vi "LIA_Host_FloatingPoint.vi"() -> ()   [LabVIEW 2012]
uses:
  <vilib>/userdefined/High Color/nirio_resource_hc.ctl
  <vilib>/LabVIEW Targets/FPGA/cRIO/shared/nicrio_ModuleControls/nicrio_cRIO-9233_DataRatesRing.ctl
  <vilib>/FPGAPlugInAG/PCI-7831R/niLvFpga_Open_PCI-7831R.vi
  <vilib>/FPGAPlugInAG/PCI-7831R/niLvFpga_Download_PCI-7831R.vi
  <vilib>/FPGAPlugInAG/PCI-7831R/niLvFpga_Reset_PCI-7831R.vi
  <vilib>/Utility/error.llb/Error Cluster From Error Code.vi
  <vilib>/FPGAPlugInAG/PCI-7831R/niLvFpga_Run_PCI-7831R.vi
  <vilib>/RVI Host/nirviSupport.llb/nirviErrorClusterFromErrorCode.vi
  <vilib>/rvi/errors/niLvFpgaAdjustHostInterfaceError.vi
  <vilib>/FPGAPlugInAG/PCI-7831R/niLvFpga_Close_PCI-7831R.vi
  <vilib>/rvi/interface/nirviOpenFPGA/nirviOpenFPGA.xnode
  FPGA Bitfiles/LIA_FPGATarget_LIAFPGA_UBXKlbf10UU.lvbitx
  LIA_FPGA.vi
  <vilib>/rvi/interface/nirviMethod/nirviMethod.xnode
  <vilib>/rvi/interface/nirviReadWriteControl/nirviReadWriteControl.xnode
  <vilib>/rvi/interface/nirviCloseFPGA/nirviCloseFPGA.xnode
  <vilib>/rvi/errors/niLvFpgaMergeErrorWithErrorCode.vi
  <vilib>/FPGAPlugInAG/PCI-7831R/niLvFpga_ConfigureFifo_PCI-7831R.vi
  <vilib>/rvi/interface/nirviMethod/StockFPGA_InlinedMethodWaitForSingleIRQ.vi
  <vilib>/FPGAPlugInAG/PCI-7831R/niLvFpga_WaitOnIrq_PCI-7831R.vi
  <vilib>/FPGAPlugInAG/PCI-7831R/niLvFpga_AcknowledgeIrq_PCI-7831R.vi
  <vilib>/FPGAPlugInAG/PCI-7831R/niLvFpga_ReadFifo_PCI-7831R.vi
  NiFpgaLv.dll
panel:
  in  "Elements Remaining":u32
  in  "Offset":sgl
  in  "LSB Weight":sgl
  out "Locked?":bool
  out "Locked Frequency [Hz]":dbl
  out "Phase [degree]":dbl
  out "Amplitude [V]":dbl
  in  "Data Rate":T1=2 items=["50.000 kS/s (NI 9233)"=2, "33.333 kS/s (NI 9233)"=3, "25.000 kS/s (NI 9233)"=34, "16.667 kS/s (NI 9233)"=35, "12.500 kS/s (NI 9233)"=36, "10.000 kS/s (NI 9233)"=37, "  8.333 kS/s (NI 9233)"=38, "  7.143 kS/s (NI 9233)"=39, "  6.250 kS/s (NI 9233)"=40, "  5.556 kS/s (NI 9233)"=41, "  5.000 kS/s (NI 9233)"=42, "  4.545 kS/s (NI 9233)"=43, "  4.167 kS/s (NI 9233)"=44, "  3.846 kS/s (NI 9233)"=45, "  3.571 kS/s (NI 9233)"=46, "  3.333 kS/s (NI 9233)"=47, "  3.125 kS/s (NI 9233)"=48, "  2.941 kS/s (NI 9233)"=49, "  2.778 kS/s (NI 9233)"=50, "  2.632 kS/s (NI 9233)"=51, "  2.500 kS/s (NI 9233)"=52, "  2.381 kS/s (NI 9233)"=53, "  2.273 kS/s (NI 9233)"=54, "  2.174 kS/s (NI 9233)"=55, "  2.083 kS/s (NI 9233)"=56, "  2.000 kS/s (NI 9233)"=57]
  out "Waveform Graph":sgl[][](graph)
  in  "stop":bool
  out "channel Q":dbl
  out "channel I":dbl
  in  "Filter Rolloff":enum16{"20 dB", "40 dB", "60 dB", "80 dB"}(ring)
  in  "Time Constant [s]":dbl=1.0 format="%.2f"
  in  "Resource Name":T2
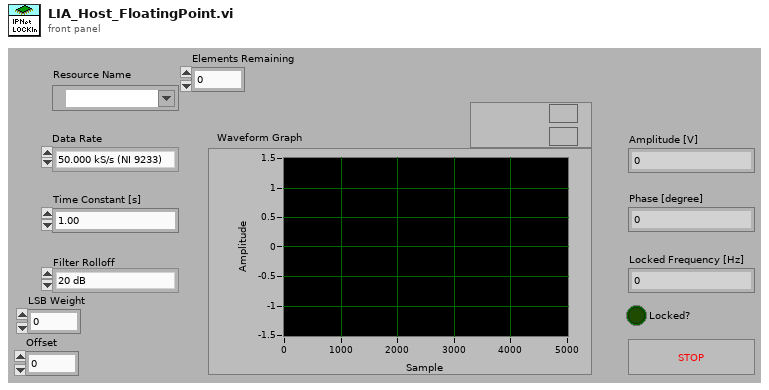
[diagram p1: front panel]
types:
  T1 = typedef "nicrio_cRIO-9233_DataRatesRing.ctl" = u8
  T2 = typedef "nirio_resource_hc.ctl" = tag
  T3 = enum16{"Reserved", "Sine", "Square", "Sine (sync)"}
  T4 = cluster{"fr":dbl, "Phase":dbl, "Order":u32, "Updated":bool, "Block Size":i32, "fs":dbl}
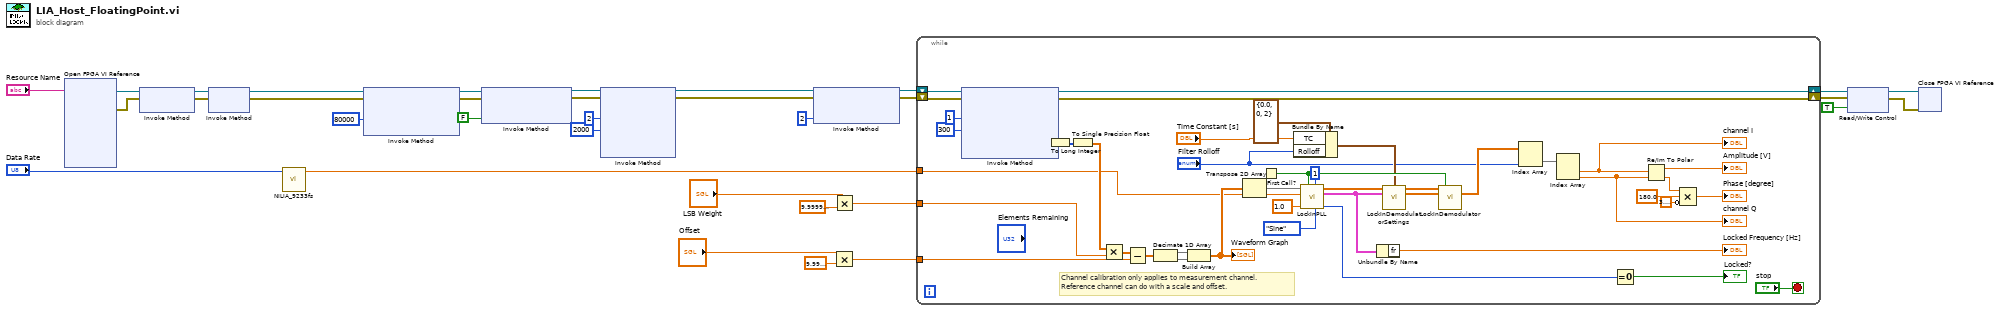
[diagram p0: block diagram]
diagram:
  n1 = xnode "Open FPGA VI Reference"("resource name"="Resource Name") -> ("FPGA VI Reference Out"=w33:refnum<k20>, "error out"=w32:errorcluster)  [unwired: 1 in]
  n2 = xnode "Invoke Method"("FPGA VI Reference In"=w33, "error in"=w32) -> ("FPGA VI Reference Out"=w31:refnum<k20>, "error out"=w30:errorcluster)
  n3 = xnode "Invoke Method"("FPGA VI Reference In"=w31, "error in"=w30) -> ("FPGA VI Reference Out"=w6:refnum<k20>, "error out"=w5:errorcluster)
  n4 = call "NILIA_9233fs.vi"("Data Rate"="Data Rate") -> ("fs"=w7:dbl)  [unwired: 10 in]
  n5 = xnode "Invoke Method"("FPGA VI Reference In"=w6, "error in"=w5, "Requested Depth"=u32 80000 ("Depth")) -> ("FPGA VI Reference Out"=w22:refnum<k20>, "error out"=w21:errorcluster)  [unwired: 1 out]
  n6 = xnode "Invoke Method"("FPGA VI Reference In"=w22, "error in"=w21, "Wait Until Done (F)"=FALSE) -> ("FPGA VI Reference Out"=w27:refnum<k20>, "error out"=w26:errorcluster)
  n7 = xnode "Invoke Method"("FPGA VI Reference In"=w27, "error in"=w26, "IRQ Number(s)"=2, "Timeout (ms)"=2000) -> ("FPGA VI Reference Out"=w2:refnum<k20>, "error out"=w1:errorcluster)  [unwired: 2 out]
  n8 = xnode "Invoke Method"("FPGA VI Reference In"=w2, "error in"=w1, "IRQ Number(s)"=2) -> ("FPGA VI Reference Out"=w20:refnum<k20>, "error out"=w19:errorcluster)
  n9 = Multiply(x="Offset", y=sgl 1e-09) -> (x*y=w9:sgl)
  n10 = Multiply(x="LSB Weight", y=sgl 1e-12) -> (x*y=w17:sgl)
  n11 = while {
    shift-right: [w62] -> w16
    shift-left: w20 -> [w70]
    shift-right: [w61] -> w15
    shift-left: w19 -> [w69]
    tunnel: w17 -> [w67]
    tunnel: w9 -> [w68]
    tunnel: w7 -> [w46]
    stop <- "stop" stop-if-true
    # "Channel calibration only applies to measurement channel.\nReference channel can do with a scale and offset."
    n12 = xnode "Invoke Method"("FPGA VI Reference In"=w70, "error in"=w69, "Number of Elements"=u32 1, "Timeout (ms)"=300) -> ("FPGA VI Reference Out"=w62:refnum<k20>, "error out"=w61:errorcluster, "Data"=w72:i32[])  [unwired: 1 out]
    n13 = To Long Integer(number=w72) -> (32bit integer=w71:i32[])
    n14 = To Single Precision Float(number=w71) -> (single precision float=w66:sgl[])
    n15 = Multiply(x=w66, y=w67) -> (x*y=w73:sgl[])
    n16 = Subtract(x=w73, y=w68) -> (x-y=w63:sgl[])
    n17 = Decimate 1D Array(w63) -> (w64:sgl[], w65:sgl[])
    n18 = Build Array(w64, w65) -> (w47:sgl[][])
    "Waveform Graph" <- w47
    n19 = Transpose 2D Array(2D array=w47) -> (transposed array=w50:sgl[][])
    n20 = First Call?() -> (First Call?: T/F=w60:bool)
    n21 = Bundle By Name(cluster=cluster{"TC":dbl, "Rolloff":u16, "Type":u16} {"TC"=0.0, "Rolloff"=0, "Type"=2} ("LP Filter Info"), "TC"="Time Constant [s]", "Rolloff"="Filter Rolloff") -> (w54:cluster{"TC":dbl, "Rolloff":u16, "Type":u16})
    n22 = call "LockInPLL.vi"("Function"=T3."Sine", "Order"=u32 1, "Init"=w60, "Filter TC (s)"=1.0, "fs"=w46, "Signal (in)"=w50) -> ("Lock error"=w34:i32, "Reference Info"=w57:T4, "Signal (out)"=w55:sgl[][])  [unwired: 2 in, 1 out]
    n23 = Unbundle By Name(w57) -> ("fr"=→"Locked Frequency [Hz]":dbl)
    n24 = call "LockInDemodulatorSettings.vi"("Signal (in)"=w55, "LP Filter Info"=w54, "Reference Info"=w57) -> ("Signal (out)"=w59:sgl[][], "LP Filter Settings"=w58:dbl[])  [unwired: 9 in, 2 out]
    n25 = call "LockInDemodulator.vi"("Signal (in)"=w59, "Apply"=w60, "LP Filter Settings"=w58) -> ("Data (out)"=w56:dbl[][])  [unwired: 10 in, 2 out]
    n26 = Index Array(array=w56, index (col)="Filter Rolloff") -> (element=w49:dbl[])  [unwired: 1 in]
    n27 = Index Array(array=w49) -> (element #1=w38:dbl, element #2=w37:dbl)  [unwired: 2 in]
    "channel I" <- w38
    "channel Q" <- w37
    n28 = Equal To 0?(x=w34) -> (x = 0?=→"Locked?":bool)
    n29 = Re/Im To Polar(2:w37, 3:w38) -> (0:w43:dbl, 1:→"Amplitude [V]":dbl)
    n30 = Compound Arithmetic op=MULTIPLY(w43, 180.0 ("value"), invert 3.141592653589793) -> (→"Phase [degree]":dbl)
  }
  n31 = xnode "Read/Write Control"("FPGA VI Reference In"=w16, "error in"=w15, "stop"=TRUE) -> ("FPGA VI Reference Out"=w13:refnum<k20>, "error out"=w12:errorcluster)
  n32 = xnode "Close FPGA VI Reference"("FPGA VI Reference In"=w13, "error in"=w12) -> ()  [unwired: 1 out]
